vi "getTaskReference.vi"(8 "error in (no error)":errorcluster, 11 "ExampleTask_StopNotifier in":refnum<class "ExampleTask_StopNotifier.lvclass">) -> (0 "error out":errorcluster, 2 "taskRef":refnum<vi>, 3 "ExampleTask_StopNotifier out":refnum<class "ExampleTask_StopNotifier.lvclass">)   [LabVIEW 2023, in "ExampleTask_StopNotifier.lvclass"]
doc: "Returns the VI reference related to the task to handle."
uses:
  ExampleTask_StopNotifier.lvclass
  ExampleTask_StopNotifier.lvclass/ExampleTask_StopNotifier.ctl
  myTask.vi
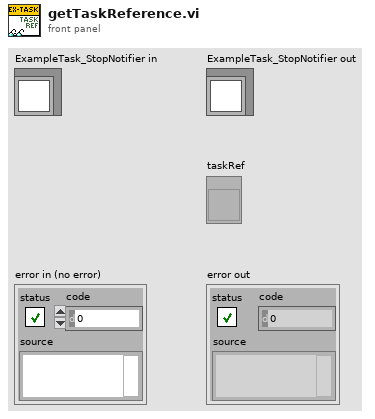
[diagram p1: front panel]
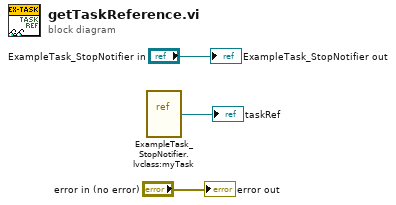
[diagram p0: block diagram]
diagram:
  n1 = vi-ref "ExampleTask_StopNotifier.lvclass:myTask.vi"() -> (→"taskRef":refnum<vi>)
  "error out" <- "error in (no error)"
  "ExampleTask_StopNotifier out" <- "ExampleTask_StopNotifier in"
